vi "lvEtherbone.VI-Tree.vi"   [LabVIEW 2012, in "lvEtherbone.lvlib"]
doc: "Contains all VIs of the LabVIEW-Etherbone interface.\n\nauthor: Dietrich Beck, GSI\nCopyright (C): GSI Helmholtzzentrum für Schwerionenforschung\nlicense: GPLv3\n\nFor details see description of lvEtherbone.lvlib"
uses:
  lvEtherbone.lvlib
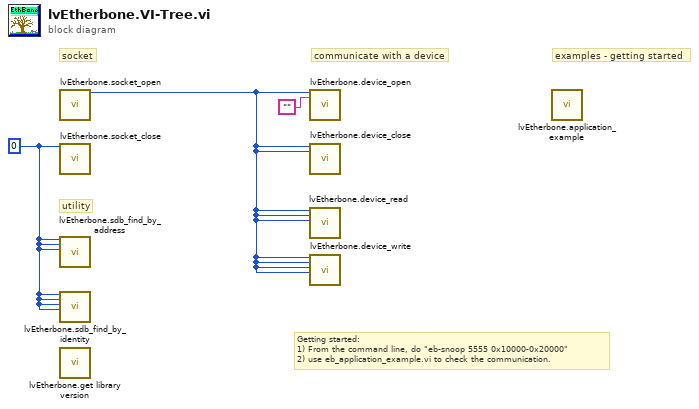
[diagram p0: block diagram]
diagram:
  w2 = 0 ("eb_socket_ID")
  # "utility"
  # "Getting started: \n1) From the command line, do \"eb-snoop 5555 0x10000-0x20000\"\n2) use eb_application_example.vi to check the communication."
  # "examples - getting started"
  # "communicate with a device"
  # "socket"
  n1 = call "lvEtherbone.socket_open.vi"() -> ("eb_socket_ID"=w1:i32)  [unwired: 17 in, 2 out]
  n2 = call "lvEtherbone.socket_close.vi"("eb_socket_ID"=w2) -> ()  [unwired: 17 in, 2 out]
  n3 = call "lvEtherbone.sdb_find_by_address.vi"("eb_socket_ID"=w2, "eb_device_ID"=w2, "address"=w2) -> ()  [unwired: 8 in, 9 out]
  n4 = call "lvEtherbone.sdb_find_by_identity.vi"("eb_socket_ID"=w2, "eb_device_ID"=w2, "vendor_id"=w2, "device_id"=w2) -> ()  [unwired: 8 in, 8 out]
  n5 = call "lvEtherbone.get library version.vi"() -> ()  [unwired: 1 in, 1 out]
  n6 = call "lvEtherbone.device_open.vi"("eb_socket_ID"=w1, "address"="" ("ip_port")) -> ()  [unwired: 14 in, 4 out]
  n7 = call "lvEtherbone.device_close.vi"("eb_socket_ID"=w1, "eb_device_ID"=w1) -> ()  [unwired: 15 in, 3 out]
  n8 = call "lvEtherbone.device_read.vi"("eb_socket_ID"=w1, "eb_device_ID"=w1, "address"=w1) -> ()  [unwired: 12 in, 5 out]
  n9 = call "lvEtherbone.device_write.vi"("eb_socket_ID"=w1, "eb_device_ID"=w1, "address"=w1, "data"=w1) -> ()  [unwired: 12 in, 4 out]
  n10 = call "lvEtherbone.application_example.vi"() -> ()  [unwired: 12 in]
